vi "Connect to Analog DAQ Example.vi"() -> ()   [LabVIEW 2018]
uses:
  Analog DAQ/Analog DAQ.lvclass
panel:
  out "Current Value":dbl format="%0.2f"
  out "error out":errorcluster
  in  "Instance Inbox Address":string
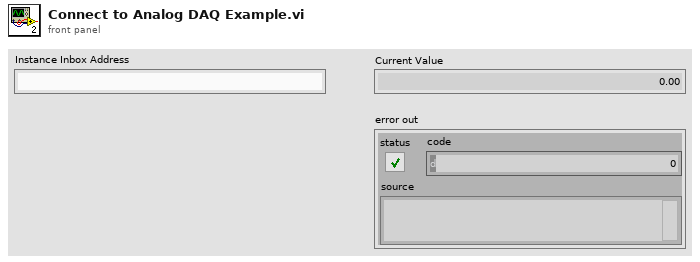
[diagram p1: front panel]
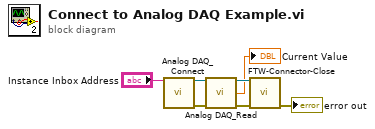
[diagram p0: block diagram]
diagram:
  n1 = call "Analog DAQ_Connect.vi"("Instance Inbox Address"="Instance Inbox Address") -> ("Analog DAQ Out"=w3:refnum<class "Analog DAQ.lvclass">, "error out"=w6:errorcluster)  [unwired: 13 in]
  n2 = call "Analog DAQ_Read.vi"("Analog DAQ In"=w3, "error in (no error)"=w6) -> ("Analog DAQ Out"=w2:refnum<class "Analog DAQ.lvclass">, "Current Value"=→"Current Value":dbl, "error out"=w4:errorcluster)  [unwired: 11 in]
  n3 = call-dynamic "FTW-Connector-Close.vi"("FTW Actor Connector"=w2, "error in"=w4) -> ("error out"=→"error out":errorcluster)  [unwired: 13 in]
